vi "Draw Donut.vi"(6 "Donut Para Array":T1[](array[typedef]), 8 "错误输入":errorcluster, 9 "Radius":i16[](array[numeric]), 10 "Center":T2, 11 "Pic in":picture) -> (0 "错误输出":errorcluster, 3 "Pic out":picture)   [LabVIEW 2011, in "Basic Shape.lvlib"]
uses:
  Basic Shape.lvlib
  Point Custom Control.ctl
  Draw Para Custom Control.ctl
panel:
  # "Array"
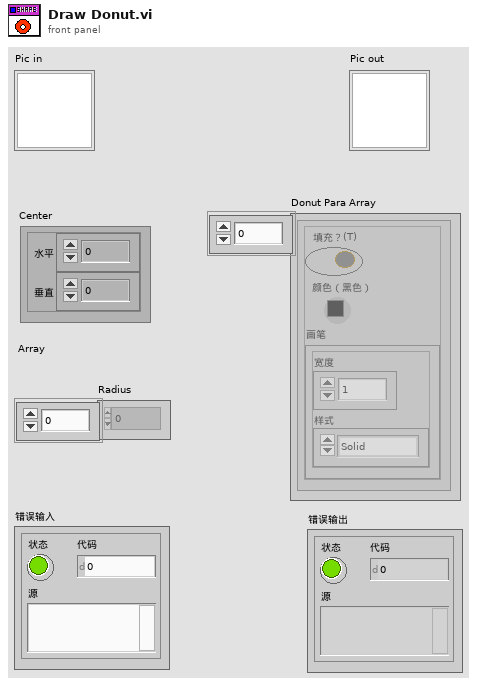
[diagram p1: front panel]
types:
  T1 = typedef "Basic Shape.lvlib/Draw Para Custom Control.ctl" = cluster{"fill?(F)":bool, "color(black)":u32, "pen":cluster{"Width":u16, "Style":enum32{"Solid", "Dash", "Dot", "DashDot", "DashDotDot"}}}
  T2 = typedef "Basic Shape.lvlib/Point Custom Control.ctl" = cluster{"horizontal":i16, "vertical":i16}
  T3 = cluster{"Width":u16, "Style":enum32{"Solid", "Dash", "Dot", "DashDot", "DashDotDot"}}
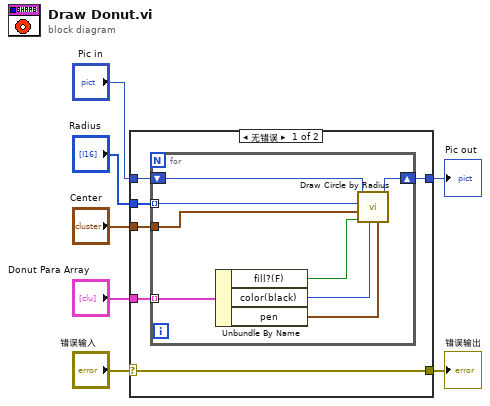
[diagram p0: block diagram]
diagram:
  n1 = case shown="无错误" "错误输入" {
    selector: "错误输入" -> [w13 w23]
    tunnel: [w13 w23] -> w6
    tunnel: "Pic in" -> [w12 w22]
    tunnel: [w11 w22] -> w4
    tunnel: "Center" -> [w10 _]
    tunnel: "Donut Para Array" -> [w9 _]
    tunnel: "Radius" -> [w8 _]
    frame No Error {
      n2 = for {
        tunnel: w9 -> [w19] mode=indexing
        shift-right: [w20] -> w11
        shift-left: w12 -> [w21]
        tunnel: w10 -> [w16]
        tunnel: w8 -> [w15] mode=indexing
        n3 = Unbundle By Name(w19) -> ("fill?(F)"=w14:bool, "color(black)"=w18:u32, "pen"=w17:T3)
        n4 = call <vilib>:"Draw Circle by Radius.vi"("pen"=w17, "color(black)"=w18, "fill?(F)"=w14, "pixel center"=w16, "radius"=w15, "picture"=w21) -> ("new picture"=w20:picture)  [unwired: 5 in]
      }
    }
    frame Error {
    }
  }
  "错误输出" <- w6
  "Pic out" <- w4
